vi "search.vi"(8 "error in (no error)":errorcluster, 10 "tag_name":string, 11 "configuration []":T1[](array[typedef])) -> (0 "error out":errorcluster, 1 "index":i32, 2 "configuration":T1={"tag_name"="", "type"="<type>", "zero"=0.0, "formula"="", "points"=[]})   [LabVIEW 2015, in "lv-calibration.lvlib"]
uses:
  lv-calibration.lvlib
  <userlib>/antonio-alexander/lv-calibration/public/_controls/configuration.ctl
  _controls/type.ctl
  <userlib>/antonio-alexander/lv-calibration/public/_controls/point.ctl
  _controls/error.ctl
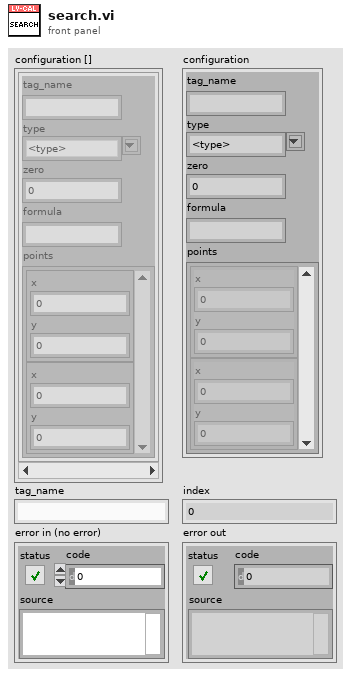
[diagram p1: front panel]
types:
  T1 = typedef "configuration.ctl" = cluster{"tag_name":string, "type":T2, "zero":dbl, "formula":string, "points":T3[]}
  T2 = typedef "lv-calibration.lvlib/type.ctl" = string
  T3 = typedef "point.ctl" = cluster{"x":dbl, "y":dbl}
  T4 = typedef "lv-calibration.lvlib/error.ctl" = enum16{"<error>", "unsupported_calibration_type", "tag_name_not_found", "duplicate_tag_names", "formula_empty"}
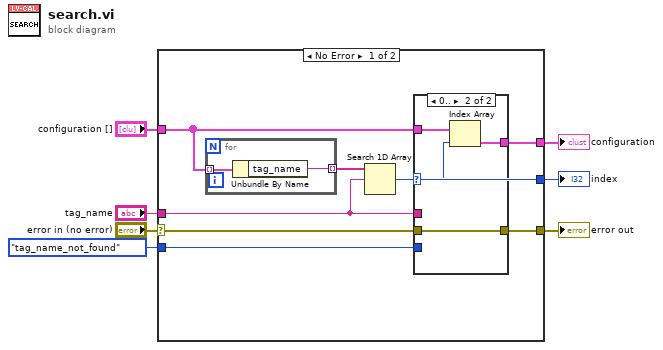
[diagram p0: block diagram]
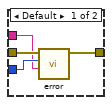
[diagram p2: hidden frame]
diagram:
  n1 = case shown="No Error" "error in (no error)" {
    selector: "error in (no error)" -> [w11 w26]
    tunnel: "configuration []" -> [w14 _]
    tunnel: [w13 _] -> w6
    tunnel: [w12 _] -> w5
    tunnel: [w10 w26] -> w3
    tunnel: error."tag_name_not_found" ("error") -> [w9 _]
    tunnel: "tag_name" -> [w8 _]
    frame No Error {
      n2 = for {
        tunnel: w14 -> [w25] mode=indexing
        tunnel: [w24] -> w15 mode=indexing
        n3 = Unbundle By Name(w25) -> ("tag_name"=w24:string)
      }
      n4 = Search 1D Array(1D array=w15, element=w8) -> (index of element=w13:i32)  [unwired: 1 in]
      n5 = case shown="0.." w13 {
        selector: w13 -> [_ w22]
        tunnel: w14 -> [_ w23]
        tunnel: [_ w21] -> w12
        tunnel: w11 -> [w19 w20]
        tunnel: [w18 w20] -> w10
        tunnel: w9 -> [w17 _]
        tunnel: w8 -> [w16 _]
        frame Default {
          n6 = call "error.vi"("data"=w16, "error"=w17, "error in (no error)"=w19) -> ("error out"=w18:errorcluster)  [unwired: 8 in]
        }
        frame 0.. {
          n7 = Index Array(array=w23, index=w22) -> (element=w21:T1)
        }
      }
    }
    frame Error {
    }
  }
  "index" <- w6
  "error out" <- w3
  "configuration" <- w5
